vi "PIMAX_2.vi"() -> ()   [LabVIEW 2018]
uses:
  <vilib>/Enthought/Python Integration Toolkit/api/Console Visibility.ctl
  Global Variables.vi
  ProgramData/Documents/Princeton Instruments/LightField/Add-in and Automation SDK/Samples/LabVIEW Automation/lightfield-automation-labview/LightField Automation.lvclass
  <vilib>/Enthought/Python Integration Toolkit/Python Integration Toolkit.lvlib
panel:
  in  "Logfile?":bool
  in  "Experiment Name":string="TestCamera"
  in  "File Path":path=path "C:/Labview Test Data/2018-10-09/UnspecifiedProj/Temp Dependence/PI_Cam1_400C"
  in  "stop":bool
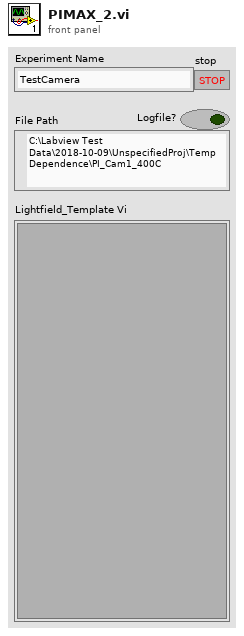
[diagram p1: front panel]
types:
  T1 = typedef "Python Integration Toolkit.lvlib/Console Visibility.ctl" = enum16{"Show Console", "Show Console While Running", "Hide Console"}
  T2 = enum32{"Bad", "Idle", "Run top level", "Running"}
  T3 = typedef "Python Integration Toolkit.lvlib/Session ID.ctl" = u64
  T4 = cluster{"Project":u16, "SubFolder":string, "Filename (Meas. Description)":string, "Measurement index":i32}
  T5 = typedef "Python Integration Toolkit.lvlib/Python Objects.ctl" = variant
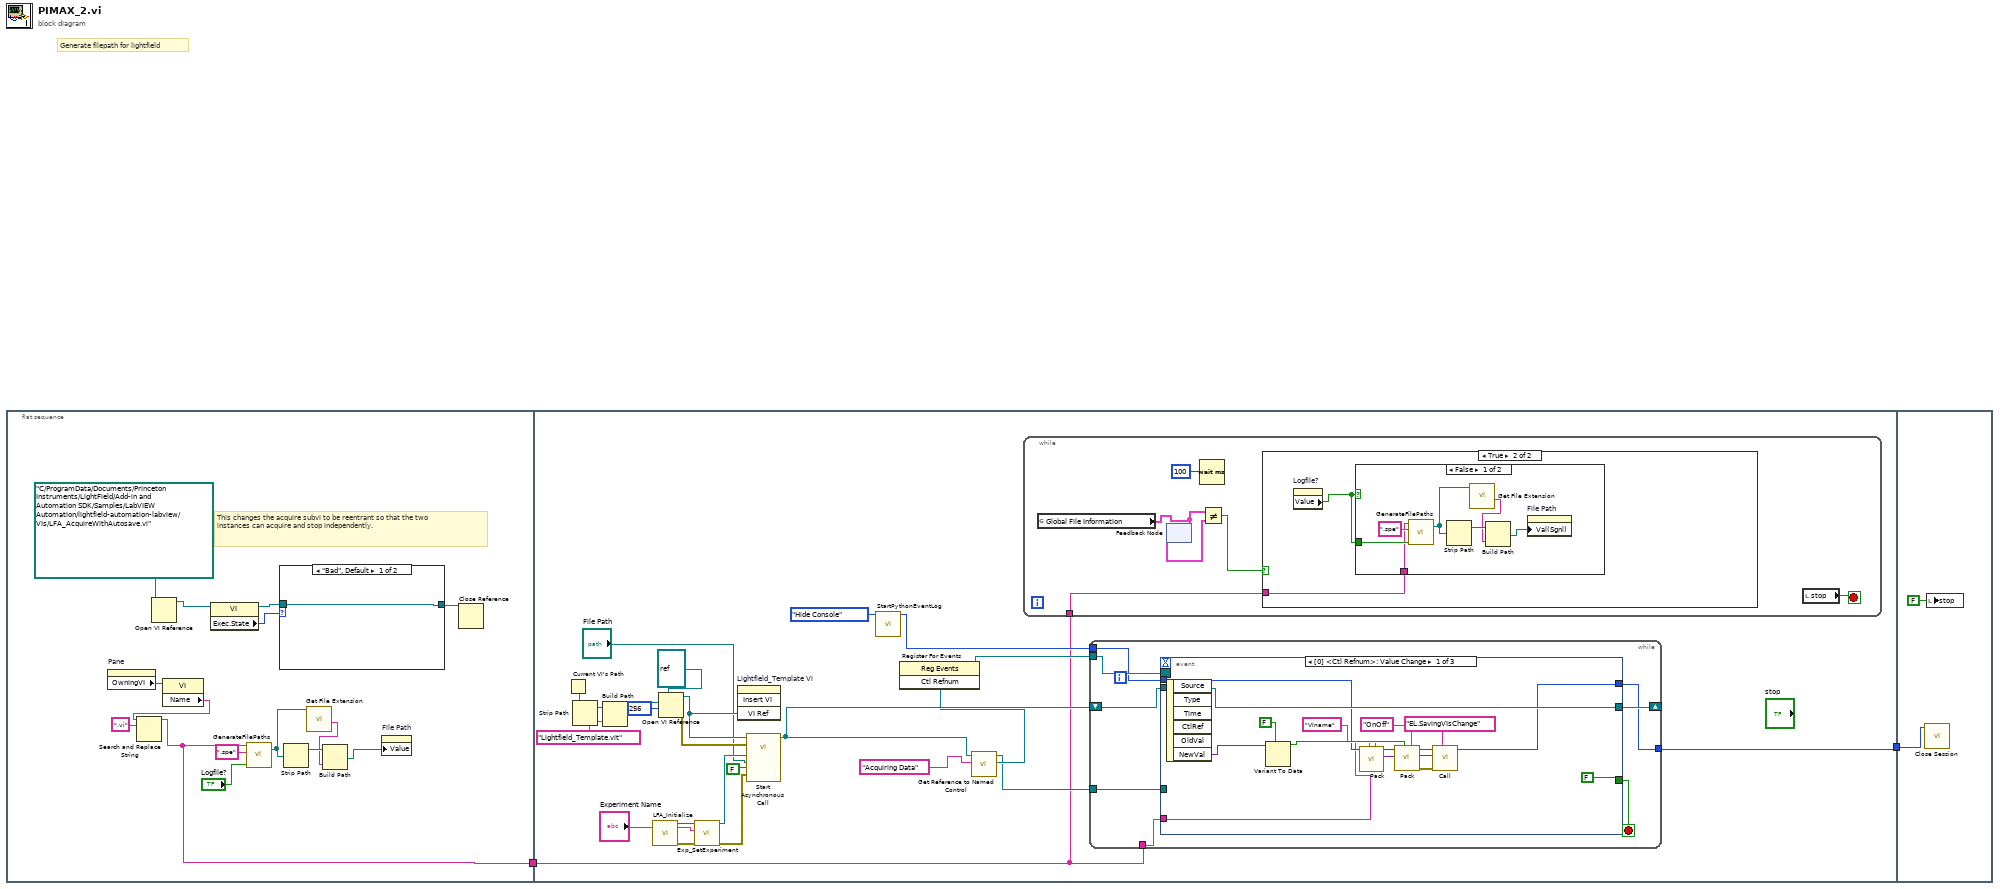
[diagram p0: block diagram]
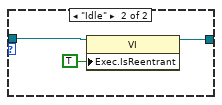
[diagram p2: hidden frame]
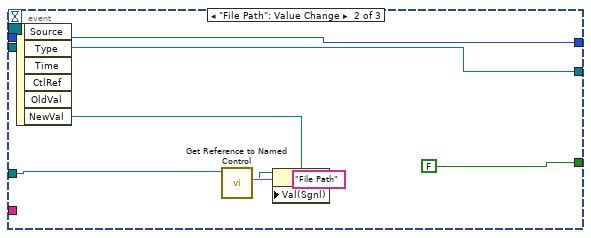
[diagram p5: hidden frame]
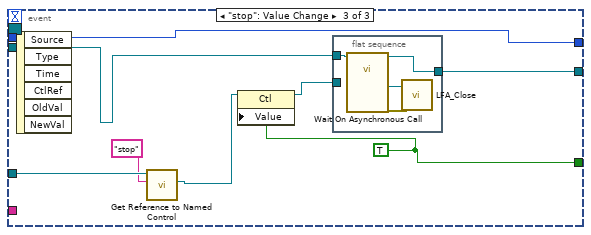
[diagram p6: hidden frame]
diagram:
  # "Generate filepath for lightfield"
  n1 = flat-sequence {
    tunnel: [w3] -> w1
    tunnel: [w29] -> w2
    tunnel: w1 -> [w22]
    tunnel: w2 -> [w104]
    frame #0 {
      # "This changes the acquire subvi to be reentrant so that the two instances can acquire and stop independently."
      n2 = property on="Pane" class="Pane"() -> ("OwningVI"=w6:refnum<vi>)  [unwired: 2 in, 2 out]
      n3 = Open VI Reference(vi path=path "C:/ProgramData/Documents/Princeton Instruments/LightField/Add-in and Automation SDK/Samples/LabVIEW Automation/lightfield-automation-labview/VIs/LFA_AcquireWithAutosave.vi") -> (vi reference=w9:refnum<vi>)  [unwired: 5 in, 1 out]
      n4 = property class="VI"(reference=w6) -> ("Name"=w4:string)  [unwired: 1 in, 2 out]
      n5 = Search and Replace String(input string=w4, search string=".vi") -> (result string=w3:string)  [unwired: 6 in, 3 out]
      n6 = property class="VI"(reference=w9) -> (reference out=w7:refnum<vi>, "Exec.State"=w8:T2)  [unwired: 1 in, 1 out]
      n7 = call "GenerateFilePaths.vi"("Logfile?"="Logfile?", "Extension (.tdms)"=".spe" ("Extension"), "Device Name"=w3) -> ("Path"=w13:path)  [unwired: 2 in]
      n8 = case shown="\"Bad\", Default" w8 {
        tunnel: [w18 w20] -> w16
        tunnel: w7 -> [w18 w19]
        frame "Bad", Default {
        }
        frame "Idle" {
          n9 = property class="VI"(reference=w19, "Exec.IsReentrant"=TRUE ("Execution:Is Reentrant")) -> (reference out=w20:refnum<vi>)  [unwired: 1 in, 1 out]
        }
      }
      n10 = Strip Path(path=w13) -> (stripped path=w12:path)  [unwired: 1 out]
      n11 = call <vilib>:"Get File Extension.vi"("file"=w13) -> ("filename without extension"=w11:string)  [unwired: 6 in, 4 out]
      n12 = Build Path(base path=w12, name or relative path=w11) -> (appended path=w10:path)
      n13 = property on="File Path" class="Path"("Value"=w10) -> ()  [unwired: 2 in, 2 out]
      n14 = Close Reference(reference=w16) -> ()  [unwired: 1 in, 1 out]
    }
    frame #1 {
      n15 = Current VI's Path() -> (path=w42:path)
      n16 = Strip Path(path=w42) -> (stripped path=w43:path)  [unwired: 1 out]
      n17 = Build Path(base path=w43, name or relative path="Lightfield_Template.vit") -> (appended path=w39:path)
      n18 = call "LFA_Initialize.vi"() -> ("error out"=w45:errorcluster, "LightField Automation out"=w44:refnum<class "LightField Automation.lvclass">)  [unwired: 10 in]
      n19 = Open VI Reference(type specifier VI Refnum (for type only)=refnum<vi> refnum, vi path=w39, options=256) -> (vi reference=w37:refnum<vi>, error out=w36:errorcluster)  [unwired: 1 in, 2 out]
      n20 = call "Exp_SetExperiment.vi"("error in (no error)"=w45, "ExperimentName"="Experiment Name", "LightField Automation in"=w44) -> ("error out"=w35:errorcluster, "LightField Automation out"=w34:refnum<class "LightField Automation.lvclass">)  [unwired: 7 in]
      n21 = invoke on="Lightfield_Template Vi" class="SubPnl" method="Insert VI"("VI Ref"=w37) -> ()  [unwired: 3 in, 4 out]
      n22 = call-by-ref "Start Asynchronous Call"(reference=w37, error in=w36, "error out"=w35, "Single Run"=FALSE, "Filepath"="File Path", "LightField Automation in"=w34) -> (reference out=w28:refnum<vi>)  [unwired: 6 in, 3 out]
      n23 = call "StartPythonEventLog.vi"("Console Visibility"=Console_Visibility."Hide Console") -> ("Session ID out"=w30:T3)  [unwired: 10 in]
      n24 = call "Get Reference to Named Control.vi"("Control Name"="Acquiring Data" ("element"), "Front Panel Ref"=w28) -> ("Ctl Refnum"=w26:refnum<vi>, "Panel Ref Out"=w25:refnum<vi>)  [unwired: 7 in, 1 out]
      n25 = register-events(w26) -> (reference out=w31:refnum<event-registration>)  [unwired: 2 in, 1 out]
      n26 = while {
        tunnel: w22 -> [w46]
        stop <- w51 stop-if-true
        n27 = global read "Global Variables.vi" "Global File Information"() -> (w49:T4)
        n28 = feedback #1() -> (w48:T4)  [unwired: 1 in]
        n29 = feedback-in #1(w49) -> ()
        n30 = Wait (ms)(milliseconds to wait=100) -> ()  [unwired: 1 out]
        n31 = Not Equal?(x=w49, y=w48) -> (x != y?=w47:bool)
        n32 = case shown="True" w47 {
          tunnel: w46 -> [_ w52]
          frame False {
          }
          frame True {
            n33 = property on="Logfile?" class="Bool (strict)"() -> ("Value"=w53:bool)  [unwired: 2 in, 2 out]
            n34 = case shown="False" w53 {
              tunnel: w53 -> [w56 _]
              tunnel: w52 -> [w54 _]
              frame False {
                n35 = call "GenerateFilePaths.vi"("Logfile?"=w56, "Extension (.tdms)"=".spe" ("Extension"), "Device Name"=w54) -> ("Path"=w59:path)  [unwired: 2 in]
                n36 = Strip Path(path=w59) -> (stripped path=w58:path)  [unwired: 1 out]
                n37 = call <vilib>:"Get File Extension.vi"("file"=w59) -> ("filename without extension"=w57:string)  [unwired: 6 in, 4 out]
                n38 = Build Path(base path=w58, name or relative path=w57) -> (appended path=w55:path)
                n39 = property on="File Path" class="Path"("Val(Sgnl)"=w55) -> ()  [unwired: 2 in, 2 out]
              }
              frame True {
              }
            }
          }
        }
        n40 = local read "stop"() -> (w51:bool)
      }
      n41 = while {
        shift-right: [w66] -> _
        shift-left: w28 -> [w67]
        tunnel: w31 -> [w65]
        tunnel: w30 -> [w64]
        tunnel: [w63] -> w29
        tunnel: w25 -> [w62]
        tunnel: w22 -> [w61]
        stop <- w68 stop-if-true
        n42 = event shown="[0] <Ctl Refnum>: Value Change" {
          selector: w65 -> [_ _ _]
          dyn-events: _ -> [_ _ _]
          timeout: _ -> [_ _ _]
          tunnel: [FALSE FALSE w99] -> w68
          tunnel: w67 -> [w83 w89 w98]
          tunnel: [w83 w89 w97] -> w66
          tunnel: w64 -> [w77 w85 w92]
          tunnel: [w70 w85 w92] -> w63
          tunnel: w62 -> [_ w87 w95]
          tunnel: w61 -> [w69 _ _]
          event Value Change {
            n43 = event-data() -> ("NewVal"=w82:variant)  [unwired: 1 in, 5 out]
            n44 = Variant To Data(type=FALSE, Variant=w82) -> (data=w80:bool)  [unwired: 1 in, 1 out]
            n45 = call <vilib>:"Pack.vi"("Keyword Name"="VIname", "Argument"=w69, "Session ID"=w77) -> ("Python Object References Out"=w72:T5, "Session ID out"=w76:T3)  [unwired: 6 in, 1 out]
            n46 = call <vilib>:"Pack.vi"("Keyword Name"="OnOff", "Argument"=w80, "Python Object References In"=w72, "Session ID"=w76) -> ("error out"=w75:errorcluster, "Python Object References Out"=w74:T5, "Session ID out"=w73:T3)  [unwired: 5 in]
            n47 = call <vilib>:"Call.vi"("Function or Method Name"="EL.SavingVIsChange", "error in (no error)"=w75, "Python Object References In"=w74, "Session ID"=w73) -> ("Session ID out"=w70:T3)  [unwired: 5 in, 2 out]
          }
          event "File Path": Value Change {
            n48 = event-data() -> ("NewVal"=w91:path)  [unwired: 1 in, 5 out]
            n49 = call "Get Reference to Named Control.vi"("Control Name"="File Path" ("element"), "Front Panel Ref"=w87) -> ("Ctl Refnum"=w86:refnum<vi>)  [unwired: 7 in, 2 out]
            n50 = property class="Ctl"(reference=w86, "Val(Sgnl)"=w91) -> ()  [unwired: 1 in, 2 out]
          }
          event "stop": Value Change {
            w99 = TRUE
            n51 = event-data() -> ()  [unwired: 1 in, 6 out]
            n52 = call "Get Reference to Named Control.vi"("Control Name"="stop", "Front Panel Ref"=w95) -> ("Ctl Refnum"=w93:refnum<vi>)  [unwired: 7 in, 2 out]
            n53 = property class="Ctl"(reference=w93, "Value"=w99) -> (reference out=w96:refnum<vi>)  [unwired: 1 in, 1 out]
            n54 = flat-sequence {
              tunnel: w98 -> [w103]
              tunnel: w96 -> [_]
              tunnel: [w100] -> w97
              frame #0 {
                n55 = call-by-ref "Wait On Asynchronous Call"(reference=w103) -> (reference out=w100:refnum<vi>, "error out 2"=w101:errorcluster, "LightField Automation out"=w102:refnum<class "LightField Automation.lvclass">)  [unwired: 11 in, 1 out]
                n56 = call "LFA_Close.vi"("error in (no error)"=w101, "LightField Automation in"=w102) -> ()  [unwired: 8 in, 2 out]
              }
            }
          }
        }
      }
    }
    frame #2 {
      n57 = call <vilib>:"Close Session.vi"("Session ID"=w104) -> ()  [unwired: 10 in, 1 out]
      n58 = local write "stop"(FALSE ("stop")) -> ()
    }
  }
